vi "Set Test Finder.vi"(8 "error in (no error)":errorcluster, 11 "Execution Profiler In":refnum<class "Execution Profiler.lvclass">) -> (0 "error out":errorcluster, 3 "Execution Profiler Out":refnum<class "Execution Profiler.lvclass">)   [LabVIEW 2020, in "Execution Profiler.lvclass"]
uses:
  Execution Profiler.lvclass
  C:/Git/astemes-lunit/source/Application Framework/Process Classes/Process/Process.lvclass
  Application Framework/Process Classes/Process/Process.lvclass/Process.ctl
  Execution Profiler.lvclass/Execution Profiler.ctl
  Application Framework/Process Classes/Process/Process.lvclass
  C:/Git/astemes-lunit/source/Framework/Execution Profiler/Execution Profiler.lvclass
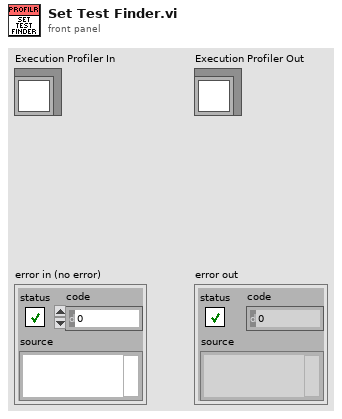
[diagram p1: front panel]
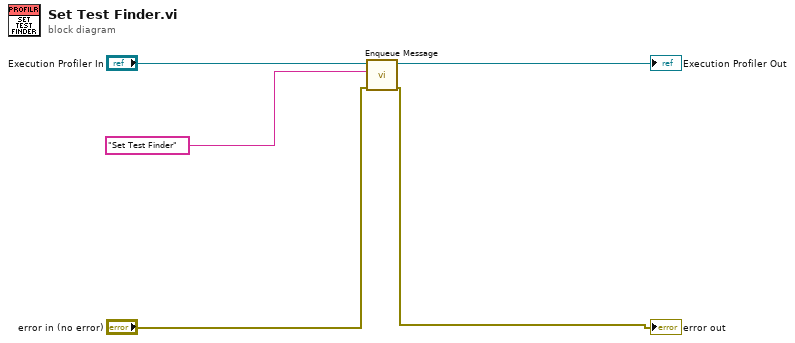
[diagram p0: block diagram]
diagram:
  n1 = call "Enqueue Message.vi"("error in (no error)"="error in (no error)", "Message"="Set Test Finder", "Process In"="Execution Profiler In") -> ("error out"=→"error out":errorcluster, "Process Out"=→"Execution Profiler Out":refnum<class "Execution Profiler.lvclass">)  [unwired: 7 in]
